vi "delete element from control by name.vi"(8 "error in":errorcluster, 10 "control label":string, 11 "VI in":refnum<vi>) -> (0 "error out":errorcluster, 3 "reference out":refnum<vi>)   [LabVIEW 2013, in "scripting tools.lvlib"]
uses:
  scripting tools.lvlib
  <vilib>/Utility/traverseref.llb/TRef TravTarget.ctl
  <vilib>/Utility/traverseref.llb/VI Scripting - Traverse.lvlib
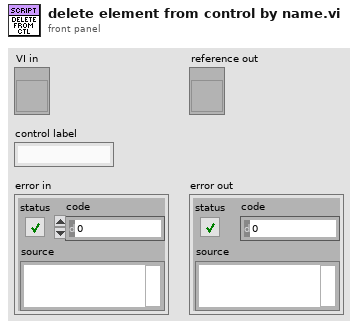
[diagram p1: front panel]
types:
  T1 = typedef "TRef TravTarget.ctl" = enum16{"FP", "BD", "Other"}
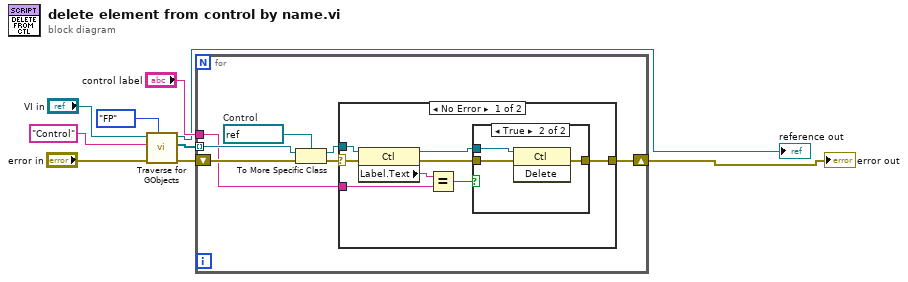
[diagram p0: block diagram]
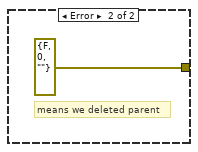
[diagram p3: hidden frame]
diagram:
  n1 = call <vilib>:"Traverse for GObjects.vi"("Traverse Target"=TRef_TravTarget."FP", "error in (no error)"="error in", "Class Name"="Control", "VI Refnum"="VI in") -> ("error out"=w5:errorcluster, "References"=w4:refnum<vi>[], "dup VI Refnum"=→"reference out":refnum<vi>)  [unwired: 4 in, 1 out]
  n2 = for {
    tunnel: w4 -> [w15] mode=indexing
    tunnel: "control label" -> [w12]
    shift-right: [w11] -> w2
    shift-left: w5 -> [w16]
    w14 = refnum<vi> refnum  # Control
    n3 = To More Specific Class(target class=w14, reference=w15, error in=w16) -> (specific class reference=w13:refnum<vi>, error out=w10:errorcluster)
    n4 = case shown="No Error" w10 {
      selector: w10 -> [w17 _]
      tunnel: w13 -> [w24 _]
      tunnel: w12 -> [w22 _]
      tunnel: [w18 errorcluster {"status"=FALSE, "code"=0, "source"=""} ("error out")] -> w11
      frame No Error {
        n5 = property class="Ctl"(reference=w24, error in=w17) -> (reference out=w19:refnum<vi>, error out=w20:errorcluster, "Label.Text"=w23:string)
        n6 = Equal?(x=w23, y=w22) -> (x = y?=w21:bool)
        n7 = case shown="True" w21 {
          tunnel: w20 -> [w25 w28]
          tunnel: w19 -> [_ w27]
          tunnel: [w25 w26] -> w18
          frame False {
          }
          frame True {
            n8 = invoke class="Ctl" method="Delete"(reference=w27, error in=w28) -> (error out=w26:errorcluster)  [unwired: 1 in, 2 out]
          }
        }
      }
      frame Error {
        # "means we deleted parent"
      }
    }
  }
  "error out" <- w2
